vi "Scan Setup.vi"(8 "error in (no error)":errorcluster, 11 "Varian Magnet Scan in":refnum<class "Varian Magnet Scan.lvclass">) -> (0 "error out":errorcluster, 3 "Varian Magnet Scan out":refnum<class "Varian Magnet Scan.lvclass">)   [LabVIEW 2009, in "Varian Magnet Scan.lvclass"]
doc: "Configure the Instrument based on the class member fields. This step comes after the user has closed the \"Scan Setup\" window and before the actual scan -- so instruments are configured with the user's specified settings."
uses:
  Varian Magnet Scan.lvclass
  Instruments/Varian Magnet/Varian Magnet.lvclass
  Scanner/Scanner.lvclass
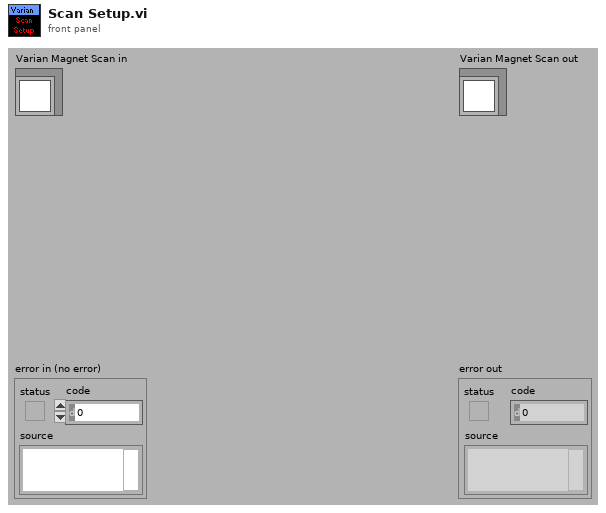
[diagram p1: front panel]
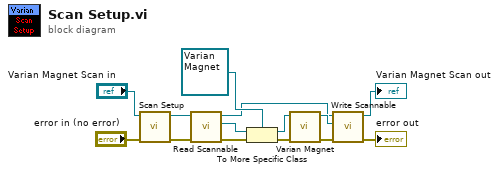
[diagram p0: block diagram]
diagram:
  n1 = call-parent "Scan Setup.vi"("error in (no error)"="error in (no error)", "Scanner in"="Varian Magnet Scan in") -> ("error out"=w12:errorcluster, "Scanner out"=w11:refnum<class "Varian Magnet Scan.lvclass">)  [unwired: 8 in]
  n2 = call-dynamic "Read Scannable.vi"("error in (no error)"=w12, "Scanner.lvclass in"=w11) -> ("error out"=w9:errorcluster, "Scannable.lvclass"=w8:refnum<class "Scannable.lvclass">, "Scanner.lvclass out"=w3:refnum<class "Varian Magnet Scan.lvclass">)  [unwired: 7 in]
  n3 = To More Specific Class(target class=refnum<class "Varian Magnet.lvclass"> refnum ("Varian Magnet.lvclass"), reference=w8, error in=w9) -> (specific class reference=w7:refnum<class "Varian Magnet.lvclass">, error out=w6:errorcluster)
  n4 = call "Varian Magnet.vi"("error in (no error)"=w6, "Varian Magnet in"=w7) -> ("error out"=w4:errorcluster, "Varian Magnet out"=w5:refnum<class "Varian Magnet.lvclass">)  [unwired: 8 in]
  n5 = call-dynamic "Write Scannable.vi"("error in (no error)"=w4, "Scannable.lvclass"=w5, "Scanner.lvclass in"=w3) -> ("error out"=→"error out":errorcluster, "Scanner.lvclass out"=→"Varian Magnet Scan out":refnum<class "Varian Magnet Scan.lvclass">)  [unwired: 7 in]
